vi "Fast Loop Controller.vi"(8 "error in":errorcluster, 9 "Fast Loop State in":T1, 11 "Fast Loop Controller in":T2) -> (0 "error out":errorcluster, 1 "Fast Loop State out":T1)   [LabVIEW 2014]
uses:
  Battery_scale.vi
  <vilib>/ptbypt/NI_PtbyPt.lvlib
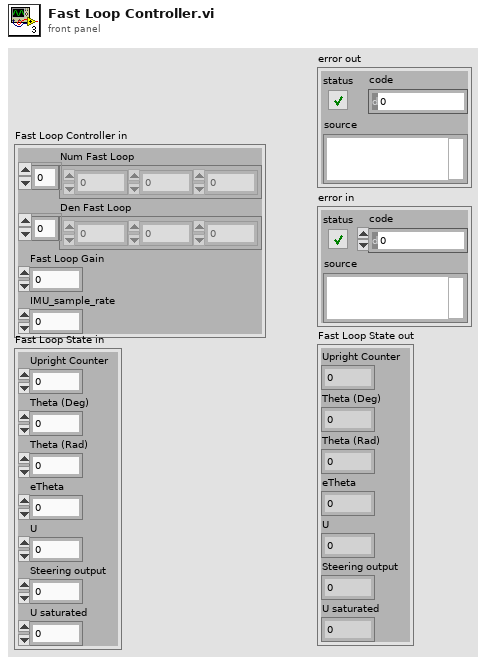
[diagram p1: front panel]
types:
  T1 = cluster{"Upright Counter":dbl, "Theta (Deg)":dbl, "Theta (Rad)":dbl, "eTheta":dbl, "U":dbl, "Steering output":dbl, "U saturated":sgl}
  T2 = cluster{"Num Fast Loop":dbl[], "Den Fast Loop":dbl[], "Fast Loop Gain":dbl, "IMU_sample_rate":i32}
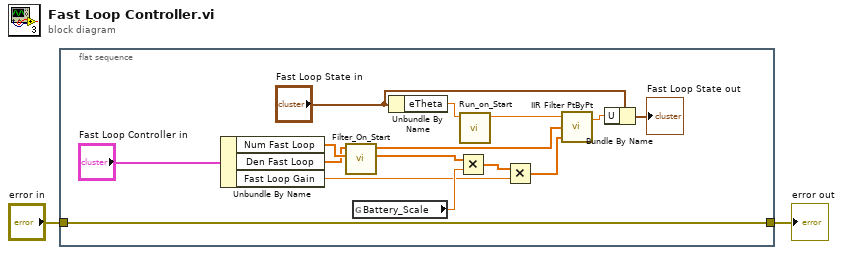
[diagram p0: block diagram]
diagram:
  n1 = flat-sequence {
    tunnel: [w12] -> w2
    tunnel: "error in" -> [w12]
    frame #0 {
      n2 = Unbundle By Name("Fast Loop Controller in") -> ("Num Fast Loop"=w10:dbl[], "Den Fast Loop"=w9:dbl[], "Fast Loop Gain"=w8:dbl)
      n3 = call "Filter_On_Start.vi"("Num In"=w10, "Denom In"=w9) -> ("Num out"=w15:dbl[], "Denom Out"=w13:dbl[])  [unwired: 8 in]
      n4 = global read "Battery_scale.vi" "Battery_Scale"() -> (w14:dbl)
      n5 = Unbundle By Name("Fast Loop State in") -> ("eTheta"=w6:dbl)
      n6 = Multiply(x=w15, y=w14) -> (x*y=w16:dbl[])
      n7 = call "Run_on_Start.vi"("val in"=w6) -> ("Val out"=w7:sgl)  [unwired: 10 in]
      n8 = Multiply(x=w16, y=w8) -> (x*y=w17:dbl[])
      n9 = call <vilib>:"IIR Filter PtByPt.vi"("Forward Coefficients"=w17, "Reverse Coefficients"=w13, "x"=w7) -> ("Filtered x"=w4:dbl)  [unwired: 1 in, 1 out]
      n10 = Bundle By Name(cluster="Fast Loop State in", "U"=w4) -> (→"Fast Loop State out":T1)
    }
  }
  "error out" <- w2
